vi "Digital Serial Gen Cfg Popup.vi"(8 "error in (no error)":errorcluster, 11 "config file in":path caption="Configuration File") -> (0 "error out":errorcluster, 2 "digital audio protocol settings":T1, 3 "config file out":path caption="Configuration File")   [LabVIEW 2021, in "Audio Popup UI.lvlib"]
uses:
  Audio Popup UI.lvlib
  digital audio protocol/digital audio protocol settings.ctl
  <vilib>/Utility/miscctls.llb/LVPointTypeDef.ctl
  digital audio protocol/digital audio protocol controls.lvlib
panel:
  in  "channel 0 offset":u32=1
  in  "Save":bool
  in  "logic level":string(combo)="3.3 V" caption="Logic level"
  in  "master clock rate":dbl=12288000.0 caption="Master clock rate" format="%#_6pHz"
  out "Bit clock rate":dbl=3072000.0 format="%#_6pHz"
  in  "number of channels":u32=2 caption="Number of channels"
  in  "TDM":bool
  in  "RJ":bool
  in  "LJ":bool
  in  "I2S":bool
  in  "bit clock edge sync":string(combo)="Falling" caption="Bit clock edge sync"
  in  "frame clock rate":dbl=48000.0 caption="Frame clock rate" format="%#_6pHz"
  in  "data justification":string(combo)="Left Justified" caption="Data justification"
  in  "endianness":string(combo)="MSB First" caption="Endianness"
  in  "bit depth":u32=24 caption="Bit depth"
  in  "channel length":u32=32 caption="Channel length"
  in  "frame sync edge for channel 0":string(combo)="Falling" caption="Frame sync edge for Channel 0"
  # "Audio Protocol"
  # "Clock Settings"
  # "Signal Level"
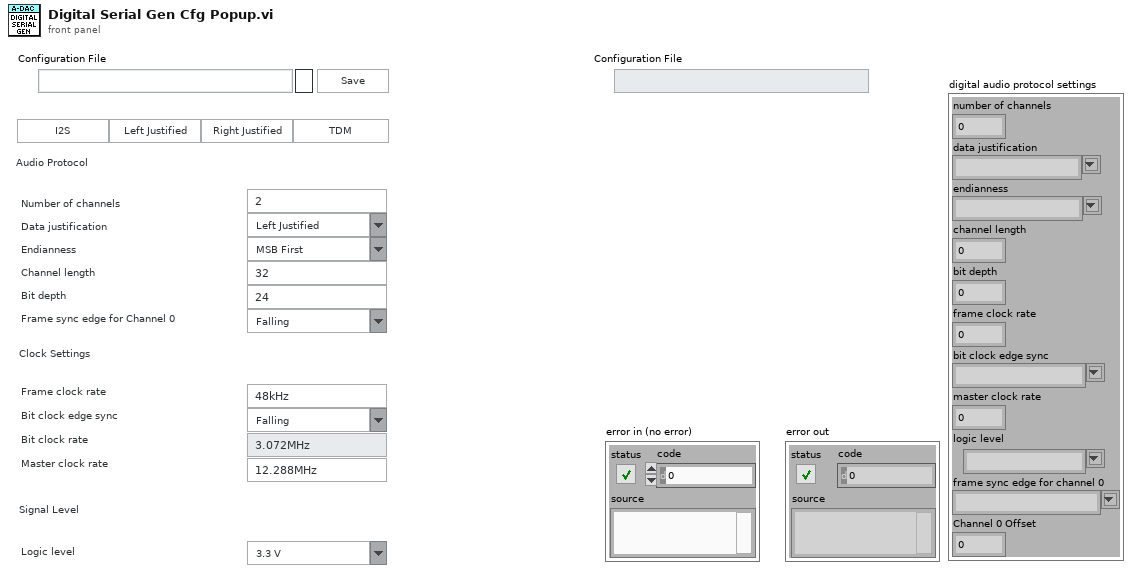
[diagram p1: front panel]
types:
  T1 = typedef "digital audio protocol controls.lvlib/digital audio protocol settings.ctl" = cluster{"number of channels":u32, "data justification":string, "endianness":string, "channel length":u32, "bit depth":u32, "frame clock rate":dbl, "bit clock edge sync":string, "master clock rate":dbl, "logic level":string, "frame sync edge for channel 0":string, "Channel 0 Offset":u32}
  T2 = typedef "LVPointTypeDef.ctl" = cluster{"Horizontal":i16, "Vertical":i16}
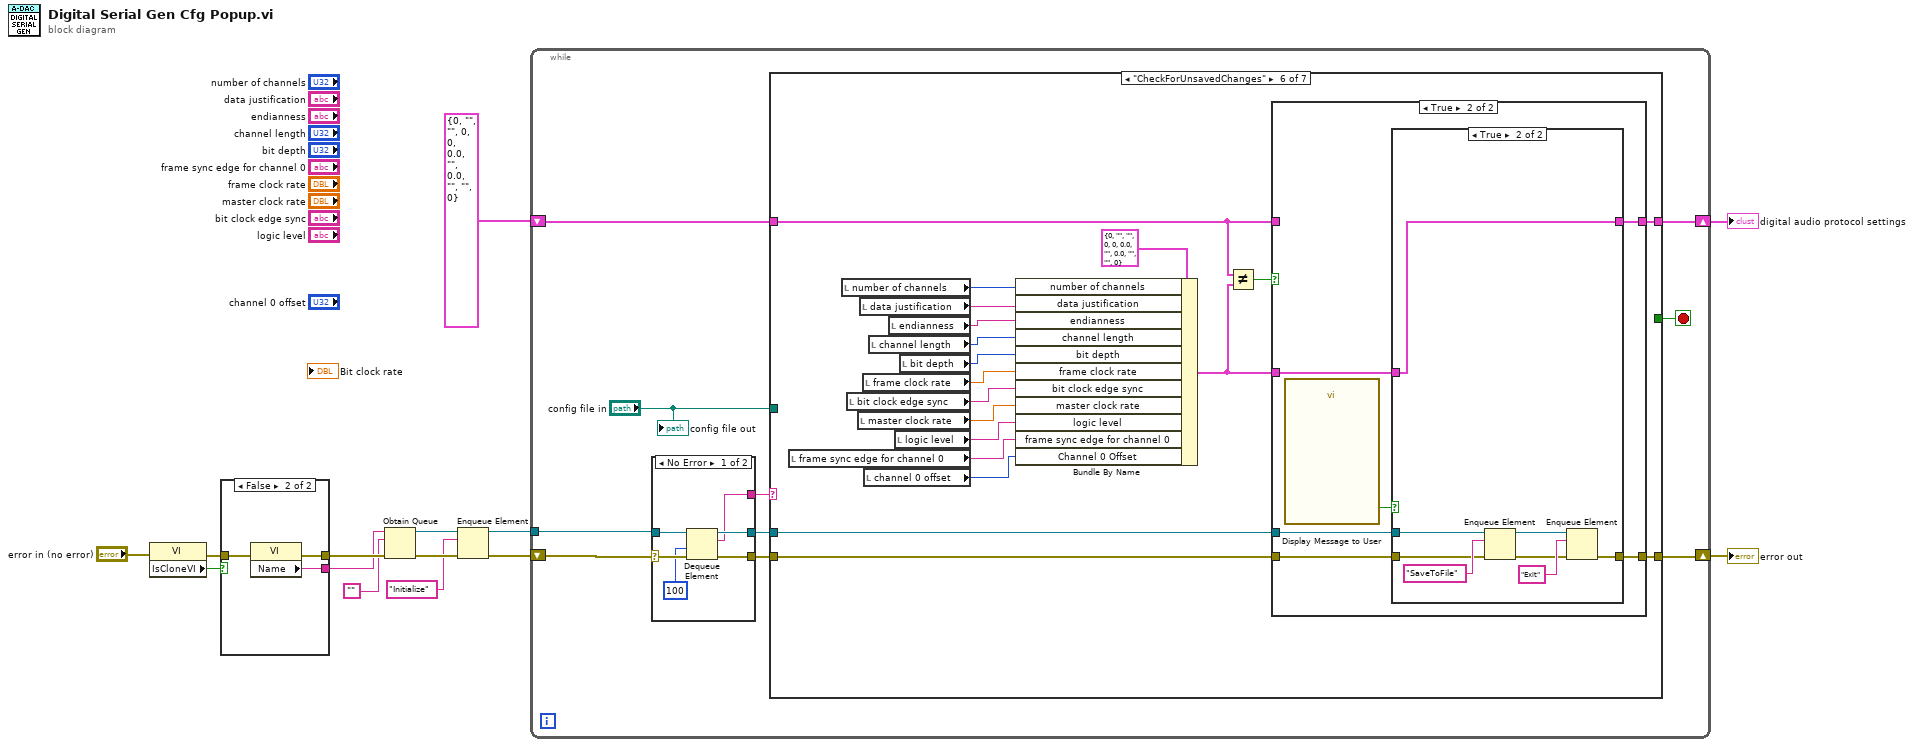
[diagram p0: block diagram]
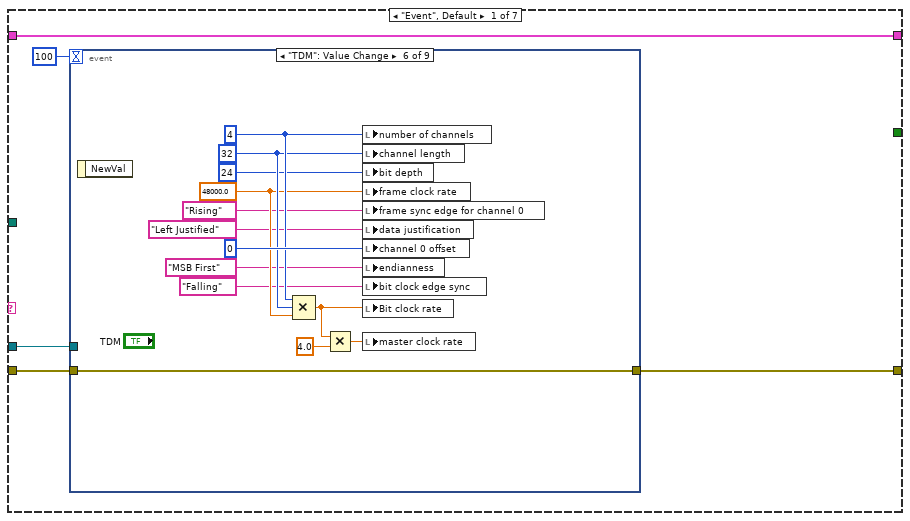
[diagram p2: hidden frame]
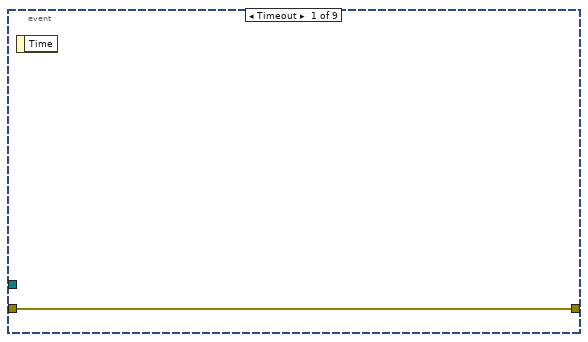
[diagram p3: hidden frame]
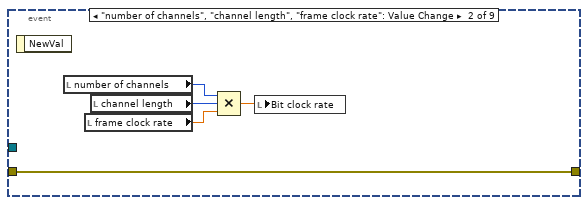
[diagram p4: hidden frame]
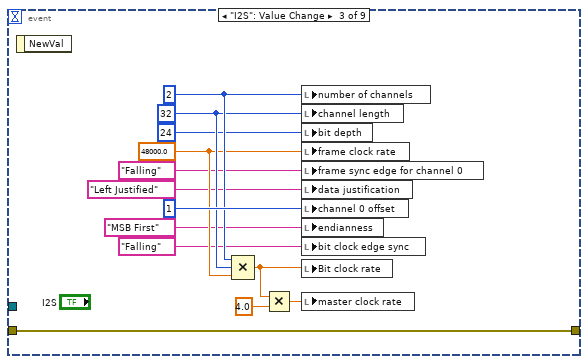
[diagram p5: hidden frame]
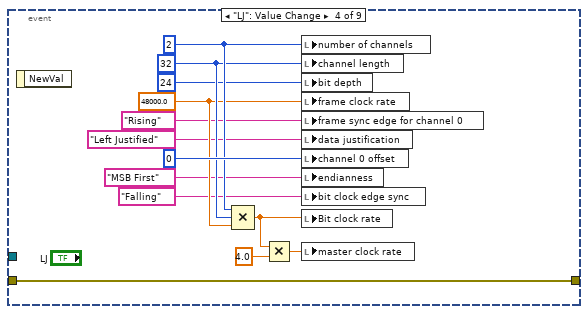
[diagram p6: hidden frame]
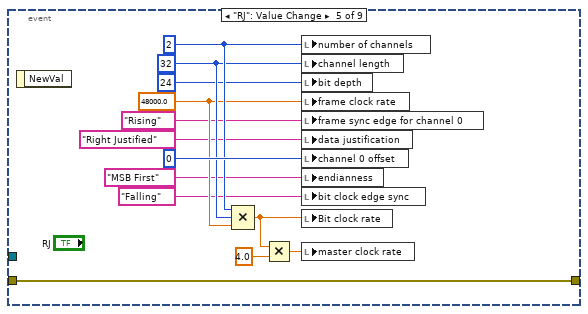
[diagram p7: hidden frame]
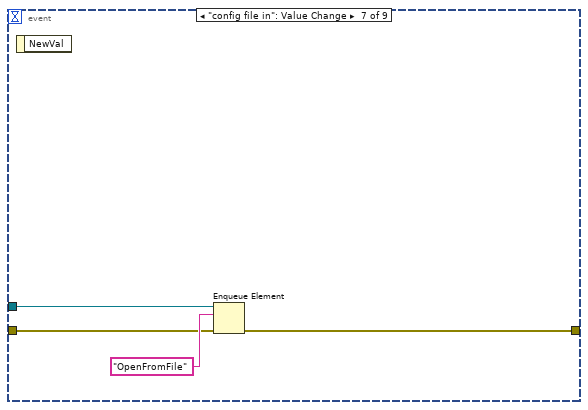
[diagram p8: hidden frame]
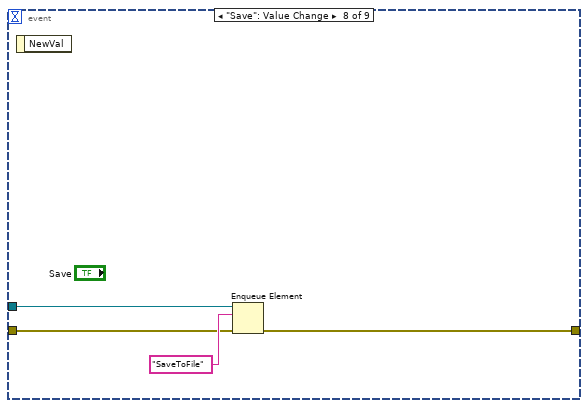
[diagram p9: hidden frame]
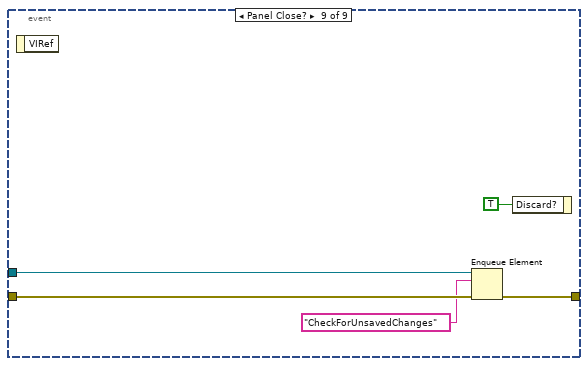
[diagram p10: hidden frame]
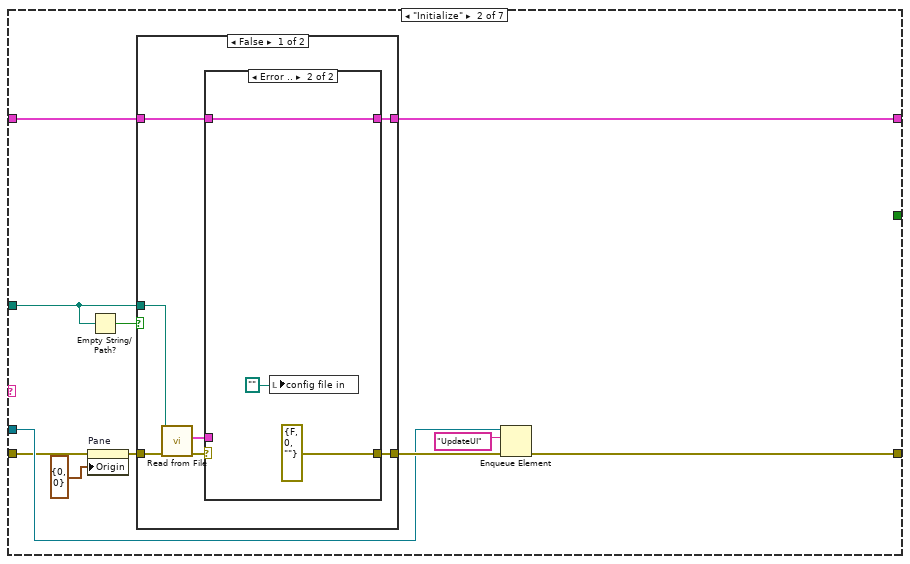
[diagram p11: hidden frame]
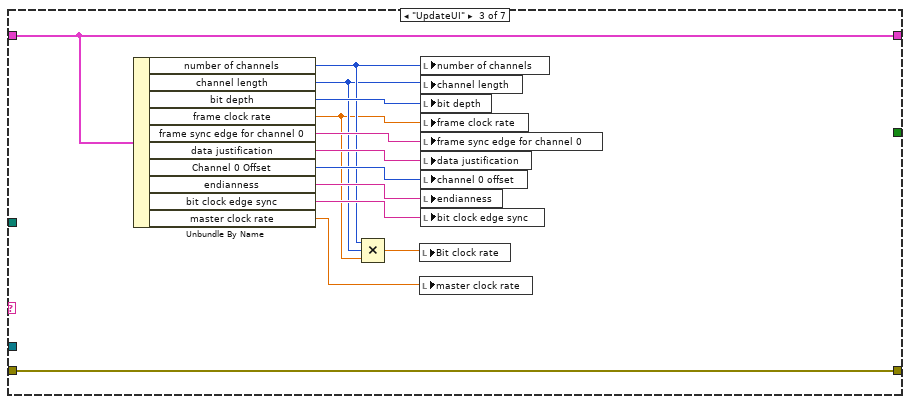
[diagram p14: hidden frame]
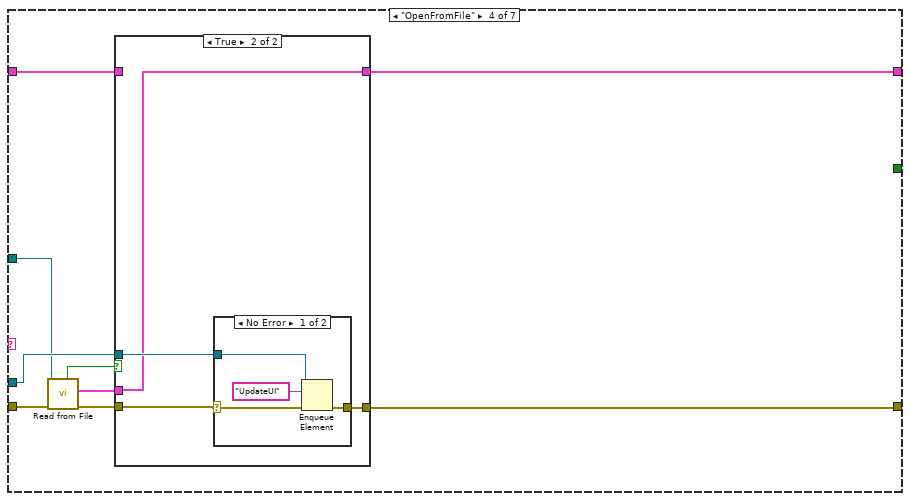
[diagram p15: hidden frame]
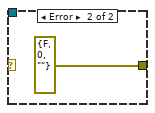
[diagram p17: hidden frame]
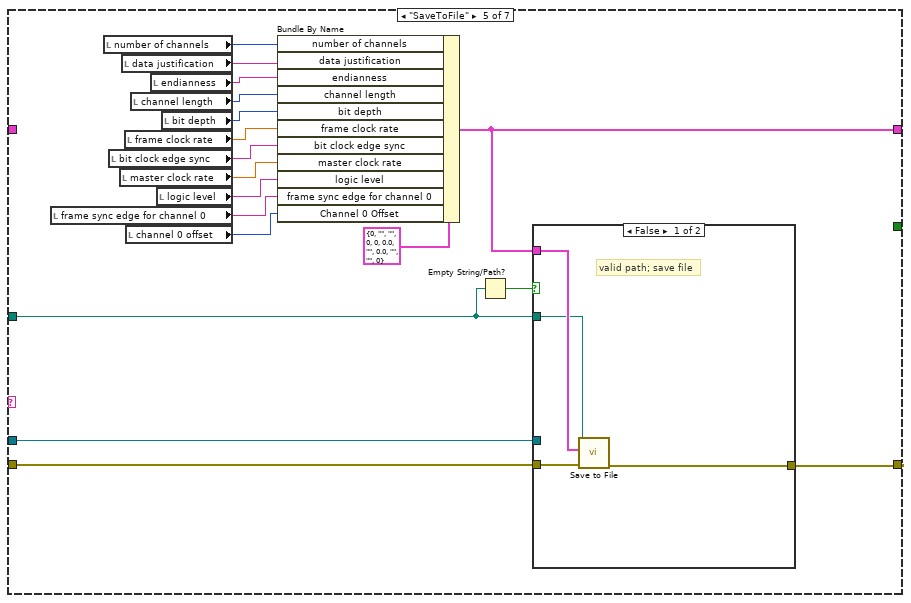
[diagram p18: hidden frame]
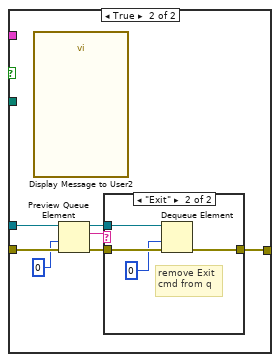
[diagram p19: hidden frame]
diagram:
  n1 = property class="VI"(error in="error in (no error)") -> (error out=w7:errorcluster, "IsCloneVI"=w8:bool)  [unwired: 1 in, 1 out]
  n2 = case shown="False" w8 {
    tunnel: [w17 w20] -> w14
    tunnel: [w16 w19] -> w13
    tunnel: w7 -> [w15 w18]
    frame True {
      n3 = property class="VI"(error in=w15) -> (error out=w17:errorcluster, "Clone Name"=w16:string)  [unwired: 1 in, 1 out]
    }
    frame False {
      n4 = property class="VI"(error in=w18) -> (error out=w20:errorcluster, "Name"=w19:string)  [unwired: 1 in, 1 out]
    }
  }
  n5 = Obtain Queue(name (unnamed)=w13, element data type="", error in (no error)=w14) -> (queue out=w11:refnum<queue>, error out=w12:errorcluster)  [unwired: 2 in, 1 out]
  n6 = Enqueue Element(queue=w11, element="Initialize", error in (no error)=w12) -> (queue out=w5:refnum<queue>, error out=w6:errorcluster)  [unwired: 1 in, 1 out]
  n7 = while {
    tunnel: w5 -> [w29]
    shift-right: [w25] -> w3
    shift-left: w6 -> [w30]
    shift-right: [w22] -> w1
    shift-left: T1 {"number of channels"=0, "data justification"="", "endianness"="", "channel length"=0, "bit depth"=0, "frame clock rate"=0.0, "bit clock edge sync"="", "master clock rate"=0.0, "logic level"="", "frame sync edge for channel 0"="", "Channel 0 Offset"=0} ("digital audio protocol settings") -> [w23]
    stop <- w24 stop-if-true
    n8 = case shown="No Error" w30 {
      selector: w30 -> [w254 w257]
      tunnel: [w253 w257] -> w26
      tunnel: w29 -> [w252 w256]
      tunnel: [w251 w256] -> w27
      tunnel: [w250 "Handle Error"] -> w28
      frame No Error {
        n9 = Dequeue Element(queue=w252, timeout in ms (-1)=100, error in (no error)=w254) -> (queue out=w251:refnum<queue>, element=w250:string, error out=w253:errorcluster)  [unwired: 1 out]
      }
      frame Error {
      }
    }
    n10 = case shown="\"CheckForUnsavedChanges\"" w28 {
      tunnel: w27 -> [w33 w112 _ w153 w165 w201 w244]
      tunnel: w26 -> [w34 w110 w144 w150 w167 w204 w245]
      tunnel: [w32 w113 w144 w152 w170 w203 w242] -> w25
      tunnel: [_ _ _ _ _ _ TRUE] -> w24
      tunnel: w23 -> [w31 w107 w143 w147 _ w199 w241]
      tunnel: [w31 w108 w143 w146 w169 w202 w241] -> w22
      tunnel: "config file in" -> [_ w116 _ w151 w168 _ _]
      frame "Event", Default {
        n11 = event shown="[5] \"TDM\": Value Change" {
          selector: _ -> [_ _ _ _ _ _ _ _ _]
          dyn-events: _ -> [_ _ _ _ _ _ _ _ _]
          timeout: 100 -> [_ _ _ _ _ _ _ _ _]
          tunnel: w34 -> [w36 w37 w46 w59 w72 w85 w96 w100 w105]
          tunnel: w33 -> [_ _ _ _ _ _ w95 w99 w104]
          tunnel: [w36 w37 w46 w59 w72 w85 w94 w98 w103] -> w32
          event Timeout {
            n12 = event-data() -> ()  [unwired: 1 in, 1 out]
          }
          event "number of channels", "channel length", "frame clock rate": Value Change {
            n13 = event-data() -> ()  [unwired: 1 in, 1 out]
            n14 = local read "number of channels"() -> (w39:u32)
            n15 = local read "frame clock rate"() -> (w38:dbl)
            n16 = local read "channel length"() -> (w40:u32)
            n17 = Compound Arithmetic op=MULTIPLY(w39, w40, w38) -> (w41:dbl)
            n18 = local write "Bit clock rate"(w41) -> ()
          }
          event "I2S": Value Change {
            w48 = 48000.0 ("Frame Clock Rate")
            w49 = u32 32 ("Channel Length")
            w50 = u32 2 ("Number of Channels")
            n19 = event-data() -> ()  [unwired: 1 in, 1 out]
            n20 = Compound Arithmetic op=MULTIPLY(w50, w49, w48) -> (w53:dbl)
            n21 = Multiply(x=w53, y=4.0) -> (x*y=w52:dbl)
            n22 = local write "number of channels"(w50) -> ()
            n23 = local write "channel length"(w49) -> ()
            n24 = local write "bit depth"(u32 24 ("Bit Depth")) -> ()
            n25 = local write "frame clock rate"(w48) -> ()
            n26 = local write "frame sync edge for channel 0"("Falling" ("frame sync edge for channel 0")) -> ()
            n27 = local write "data justification"("Left Justified" ("data justification")) -> ()
            n28 = local write "channel 0 offset"(u32 1 ("Channel 0 Offset")) -> ()
            n29 = local write "endianness"("MSB First" ("endianness")) -> ()
            n30 = local write "bit clock edge sync"("Falling" ("frame sync edge for channel 0")) -> ()
            n31 = local write "Bit clock rate"(w53) -> ()
            n32 = local write "master clock rate"(w52) -> ()
          }
          event "LJ": Value Change {
            w61 = 48000.0 ("Frame Clock Rate")
            w62 = u32 32 ("Channel Length")
            w63 = u32 2 ("Number of Channels")
            n33 = event-data() -> ()  [unwired: 1 in, 1 out]
            n34 = Compound Arithmetic op=MULTIPLY(w63, w62, w61) -> (w66:dbl)
            n35 = Multiply(x=w66, y=4.0) -> (x*y=w65:dbl)
            n36 = local write "number of channels"(w63) -> ()
            n37 = local write "channel length"(w62) -> ()
            n38 = local write "bit depth"(u32 24 ("Bit Depth")) -> ()
            n39 = local write "frame clock rate"(w61) -> ()
            n40 = local write "frame sync edge for channel 0"("Rising" ("frame sync edge for channel 0")) -> ()
            n41 = local write "data justification"("Left Justified" ("data justification")) -> ()
            n42 = local write "channel 0 offset"(u32 0 ("Channel 0 Offset")) -> ()
            n43 = local write "endianness"("MSB First" ("endianness")) -> ()
            n44 = local write "bit clock edge sync"("Falling" ("frame sync edge for channel 0")) -> ()
            n45 = local write "Bit clock rate"(w66) -> ()
            n46 = local write "master clock rate"(w65) -> ()
          }
          event "RJ": Value Change {
            w74 = 48000.0 ("Frame Clock Rate")
            w75 = u32 32 ("Channel Length")
            w76 = u32 2 ("Number of Channels")
            n47 = event-data() -> ()  [unwired: 1 in, 1 out]
            n48 = Compound Arithmetic op=MULTIPLY(w76, w75, w74) -> (w79:dbl)
            n49 = Multiply(x=w79, y=4.0) -> (x*y=w78:dbl)
            n50 = local write "number of channels"(w76) -> ()
            n51 = local write "channel length"(w75) -> ()
            n52 = local write "bit depth"(u32 24 ("Bit Depth")) -> ()
            n53 = local write "frame clock rate"(w74) -> ()
            n54 = local write "frame sync edge for channel 0"("Rising" ("frame sync edge for channel 0")) -> ()
            n55 = local write "data justification"("Right Justified" ("data justification")) -> ()
            n56 = local write "channel 0 offset"(u32 0 ("Channel 0 Offset")) -> ()
            n57 = local write "endianness"("MSB First" ("endianness")) -> ()
            n58 = local write "bit clock edge sync"("Falling" ("frame sync edge for channel 0")) -> ()
            n59 = local write "Bit clock rate"(w79) -> ()
            n60 = local write "master clock rate"(w78) -> ()
          }
          event "TDM": Value Change {
            w87 = 48000.0 ("Frame Clock Rate")
            w88 = u32 32 ("Channel Length")
            w89 = u32 4 ("Number of Channels")
            n61 = event-data() -> ()  [unwired: 1 in, 1 out]
            n62 = Compound Arithmetic op=MULTIPLY(w89, w88, w87) -> (w92:dbl)
            n63 = Multiply(x=w92, y=4.0) -> (x*y=w91:dbl)
            n64 = local write "number of channels"(w89) -> ()
            n65 = local write "channel length"(w88) -> ()
            n66 = local write "bit depth"(u32 24 ("Bit Depth")) -> ()
            n67 = local write "frame clock rate"(w87) -> ()
            n68 = local write "frame sync edge for channel 0"("Rising" ("frame sync edge for channel 0")) -> ()
            n69 = local write "data justification"("Left Justified" ("data justification")) -> ()
            n70 = local write "channel 0 offset"(u32 0 ("Channel 0 Offset")) -> ()
            n71 = local write "endianness"("MSB First" ("endianness")) -> ()
            n72 = local write "bit clock edge sync"("Falling" ("frame sync edge for channel 0")) -> ()
            n73 = local write "Bit clock rate"(w92) -> ()
            n74 = local write "master clock rate"(w91) -> ()
          }
          event "config file in": Value Change {
            n75 = event-data() -> ()  [unwired: 1 in, 1 out]
            n76 = Enqueue Element(queue=w95, element="OpenFromFile", error in (no error)=w96) -> (error out=w94:errorcluster)  [unwired: 1 in, 2 out]
          }
          event "Save": Value Change {
            n77 = event-data() -> ()  [unwired: 1 in, 1 out]
            n78 = Enqueue Element(queue=w99, element="SaveToFile", error in (no error)=w100) -> (error out=w98:errorcluster)  [unwired: 1 in, 2 out]
          }
          event Panel Close? {
            n79 = event-data() -> ()  [unwired: 1 in, 1 out]
            n80 = Enqueue Element(queue=w104, element="CheckForUnsavedChanges", error in (no error)=w105) -> (error out=w103:errorcluster)  [unwired: 1 in, 2 out]
            n81 = event-data("Discard?"=TRUE) -> ()  [unwired: 1 in, 1 out]
          }
        }
      }
      frame "Initialize" {
        n82 = property on="Pane" class="Pane"(error in=w110, "Origin"=T2 {"Horizontal"=0, "Vertical"=0}) -> (error out=w109:errorcluster)  [unwired: 1 in, 1 out]
        n83 = Empty String/Path?(string/path=w116) -> (empty?=w117:bool)
        n84 = case shown="False" w117 {
          tunnel: w109 -> [w124 w131]
          tunnel: w116 -> [w123 _]
          tunnel: [w119 w130] -> w108
          tunnel: [w121 w131] -> w114
          tunnel: w107 -> [w118 w130]
          frame False {
            n85 = call "Read from File.vi"("error in (no error)"=w124, "file path"=w123) -> ("error out"=w122:errorcluster, "digital audio protocol settings"=w120:T1)  [unwired: 7 in, 1 out]
            n86 = case shown="Error .." w122 {
              selector: w122 -> [w126 _]
              tunnel: [w126 errorcluster {"status"=FALSE, "code"=0, "source"=""} ("error IO")] -> w121
              tunnel: w120 -> [w125 _]
              tunnel: [w125 w129] -> w119
              tunnel: w118 -> [_ w129]
              frame No Error {
              }
              frame Error {
                n87 = local write "config file in"(path "") -> ()
              }
            }
          }
          frame True {
          }
        }
        n88 = Enqueue Element(queue=w112, element="UpdateUI", error in (no error)=w114) -> (error out=w113:errorcluster)  [unwired: 1 in, 2 out]
      }
      frame "UpdateUI" {
        n89 = Unbundle By Name(w143) -> ("number of channels"=w136:u32, "channel length"=w135:u32, "bit depth"=w142:u32, "frame clock rate"=w134:dbl, "frame sync edge for channel 0"=w141:string, "data justification"=w140:string, "Channel 0 Offset"=w139:u32, "endianness"=w138:string, "bit clock edge sync"=w137:string, "master clock rate"=w132:dbl)
        n90 = Compound Arithmetic op=MULTIPLY(w136, w135, w134) -> (w133:dbl)
        n91 = local write "Bit clock rate"(w133) -> ()
        n92 = local write "master clock rate"(w132) -> ()
        n93 = local write "number of channels"(w136) -> ()
        n94 = local write "channel length"(w135) -> ()
        n95 = local write "bit depth"(w142) -> ()
        n96 = local write "frame clock rate"(w134) -> ()
        n97 = local write "frame sync edge for channel 0"(w141) -> ()
        n98 = local write "data justification"(w140) -> ()
        n99 = local write "channel 0 offset"(w139) -> ()
        n100 = local write "endianness"(w138) -> ()
        n101 = local write "bit clock edge sync"(w137) -> ()
      }
      frame "OpenFromFile" {
        n102 = call "Read from File.vi"("error in (no error)"=w150, "file path"=w151) -> ("error out"=w149:errorcluster, "digital audio protocol settings"=w145:T1, "file exists?"=w148:bool)  [unwired: 7 in]
        n103 = case shown="True" w148 {
          tunnel: w153 -> [_ w159]
          tunnel: [w154 w158] -> w152
          tunnel: w149 -> [w154 w156]
          tunnel: w147 -> [w155 _]
          tunnel: [w155 w157] -> w146
          tunnel: w145 -> [_ w157]
          frame False {
          }
          frame True {
            n104 = case shown="No Error" w156 {
              selector: w156 -> [w160 _]
              tunnel: w159 -> [w162 _]
              tunnel: [w161 errorcluster {"status"=FALSE, "code"=0, "source"=""} ("error out")] -> w158
              frame No Error {
                n105 = Enqueue Element(queue=w162, element="UpdateUI", error in (no error)=w160) -> (error out=w161:errorcluster)  [unwired: 1 in, 2 out]
              }
              frame Error {
              }
            }
          }
        }
      }
      frame "SaveToFile" {
        n106 = local read "frame sync edge for channel 0"() -> (w172:string)
        n107 = local read "number of channels"() -> (w181:u32)
        n108 = local read "bit clock edge sync"() -> (w175:string)
        n109 = local read "master clock rate"() -> (w174:dbl)
        n110 = local read "data justification"() -> (w180:string)
        n111 = local read "frame clock rate"() -> (w176:dbl)
        n112 = local read "channel 0 offset"() -> (w171:u32)
        n113 = local read "channel length"() -> (w178:u32)
        n114 = local read "endianness"() -> (w179:string)
        n115 = local read "logic level"() -> (w173:string)
        n116 = local read "bit depth"() -> (w177:u32)
        n117 = Bundle By Name(cluster=T1 {"number of channels"=0, "data justification"="", "endianness"="", "channel length"=0, "bit depth"=0, "frame clock rate"=0.0, "bit clock edge sync"="", "master clock rate"=0.0, "logic level"="", "frame sync edge for channel 0"="", "Channel 0 Offset"=0} ("input cluster"), "number of channels"=w181, "data justification"=w180, "endianness"=w179, "channel length"=w178, "bit depth"=w177, "frame clock rate"=w176, "bit clock edge sync"=w175, "master clock rate"=w174, "logic level"=w173, "frame sync edge for channel 0"=w172, "Channel 0 Offset"=w171) -> (w169:T1)
        n118 = Empty String/Path?(string/path=w168) -> (empty?=w166:bool)
        n119 = case shown="False" w166 {
          tunnel: [w186 w189] -> w170
          tunnel: w169 -> [w185 _]
          tunnel: w168 -> [w184 _]
          tunnel: w167 -> [w183 w193]
          tunnel: w165 -> [_ w192]
          frame False {
            # "valid path; save file"
            n120 = call "Save to File.vi"("error in (no error)"=w183, "digital audio protocol settings"=w185, "file path"=w184) -> ("error out"=w186:errorcluster)  [unwired: 8 in]
          }
          frame True {
            n121 = call "Display Message to User2"() -> ()  [unwired: 10 in, 2 out]
            n122 = Preview Queue Element(queue=w192, timeout in ms (-1)=0, error in (no error)=w193) -> (queue out=w191:refnum<queue>, element=w187:string, error out=w190:errorcluster)  [unwired: 1 out]
            n123 = case shown="\"Exit\"" w187 {
              tunnel: w191 -> [_ w198]
              tunnel: w190 -> [w194 w197]
              tunnel: [w194 w196] -> w189
              frame "False", Default {
              }
              frame "Exit" {
                # "remove Exit\ncmd from q"
                n124 = Dequeue Element(queue=w198, timeout in ms (-1)=0, error in (no error)=w197) -> (error out=w196:errorcluster)  [unwired: 3 out]
              }
            }
          }
        }
      }
      frame "CheckForUnsavedChanges" {
        n125 = local read "frame sync edge for channel 0"() -> (w208:string)
        n126 = local read "number of channels"() -> (w217:u32)
        n127 = local read "bit clock edge sync"() -> (w211:string)
        n128 = local read "master clock rate"() -> (w210:dbl)
        n129 = local read "data justification"() -> (w216:string)
        n130 = local read "frame clock rate"() -> (w212:dbl)
        n131 = local read "channel 0 offset"() -> (w207:u32)
        n132 = local read "channel length"() -> (w214:u32)
        n133 = local read "endianness"() -> (w215:string)
        n134 = local read "logic level"() -> (w209:string)
        n135 = local read "bit depth"() -> (w213:u32)
        n136 = Bundle By Name(cluster=T1 {"number of channels"=0, "data justification"="", "endianness"="", "channel length"=0, "bit depth"=0, "frame clock rate"=0.0, "bit clock edge sync"="", "master clock rate"=0.0, "logic level"="", "frame sync edge for channel 0"="", "Channel 0 Offset"=0} ("input cluster"), "number of channels"=w217, "data justification"=w216, "endianness"=w215, "channel length"=w214, "bit depth"=w213, "frame clock rate"=w212, "bit clock edge sync"=w211, "master clock rate"=w210, "logic level"=w209, "frame sync edge for channel 0"=w208, "Channel 0 Offset"=w207) -> (w200:T1)
        n137 = Not Equal?(x=w199, y=w200) -> (x != y?=w205:bool)
        n138 = case shown="True" w205 {
          tunnel: w204 -> [w220 w228]
          tunnel: [w218 w224] -> w203
          tunnel: w200 -> [_ w226]
          tunnel: w199 -> [w222 _]
          tunnel: [w222 w225] -> w202
          tunnel: w201 -> [w219 w223]
          frame False {
            n139 = Enqueue Element(queue=w219, element="Exit", error in (no error)=w220) -> (error out=w218:errorcluster)  [unwired: 1 in, 2 out]
          }
          frame True {
            n140 = call "Display Message to User"() -> ("Yes"=w227:bool)  [unwired: 10 in, 1 out]
            n141 = case shown="True" w227 {
              tunnel: w228 -> [w232 w239]
              tunnel: w226 -> [_ w238]
              tunnel: [_ w238] -> w225
              tunnel: [w230 w234] -> w224
              tunnel: w223 -> [w231 w233]
              frame False {
                n142 = Enqueue Element(queue=w231, element="Exit", error in (no error)=w232) -> (error out=w230:errorcluster)  [unwired: 1 in, 2 out]
              }
              frame True {
                n143 = Enqueue Element(queue=w233, element="SaveToFile", error in (no error)=w239) -> (queue out=w235:refnum<queue>, error out=w236:errorcluster)  [unwired: 1 in, 1 out]
                n144 = Enqueue Element(queue=w235, element="Exit", error in (no error)=w236) -> (error out=w234:errorcluster)  [unwired: 1 in, 2 out]
              }
            }
          }
        }
      }
      frame "Exit" {
        n145 = Flush Queue(queue=w244, error in (no error)=w245) -> (queue out=w248:refnum<queue>, error out=w247:errorcluster)  [unwired: 1 out]
        n146 = Release Queue(queue=w248, force destroy? (F)=TRUE, error in (no error)=w247) -> (error out=w242:errorcluster)  [unwired: 2 out]
      }
    }
    "config file out" <- "config file in"
  }
  "error out" <- w3
  "digital audio protocol settings" <- w1
